vi "anglecalcs.vi"() -> ()   [LabVIEW 2015]
panel:
  out "thi6":dbl
  out "thi5":dbl
  out "thi4":dbl
  out "hyp2":dbl
  out "hyp1":dbl
  out "thi3":dbl
  out "thi2":dbl
  out "thi1":dbl
  out "h2":dbl
  out "h1":dbl
  out "x2":dbl
  out "x1":dbl
  in  "start":dbl[](array[numeric])
  in  "Finish":dbl[](array[numeric])
  in  "laser":dbl[](array[numeric])
  in  "laser height":dbl
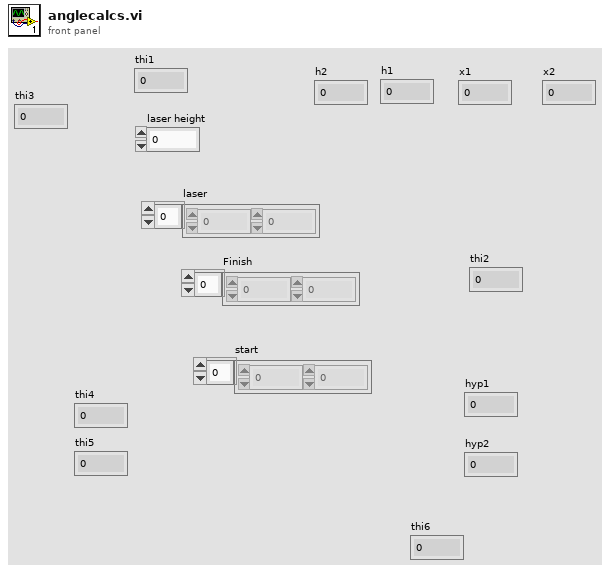
[diagram p1: front panel]
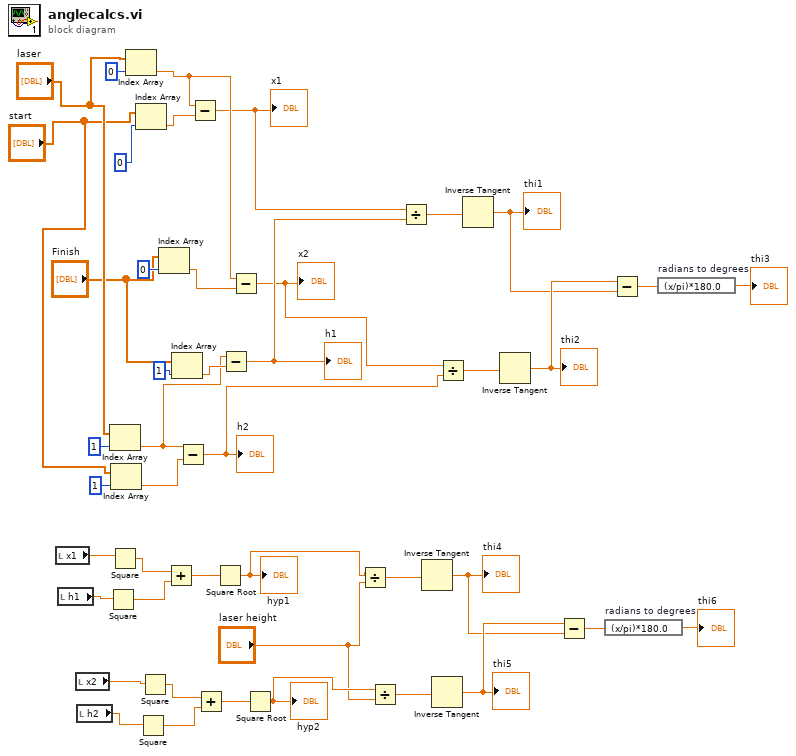
[diagram p0: block diagram]
diagram:
  n1 = local read "x1"() -> (w18:dbl)
  n2 = local read "h1"() -> (w19:dbl)
  n3 = local read "x2"() -> (w11:dbl)
  n4 = local read "h2"() -> (w10:dbl)
  n5 = Square(x=w19) -> (x^2=w16:dbl)
  n6 = Index Array(array="laser", index=1) -> (element=w30:dbl)
  n7 = Square(x=w18) -> (x^2=w17:dbl)
  n8 = Index Array(array="start", index=1) -> (element=w33:dbl)
  n9 = Index Array(array="laser", index=0) -> (element=w41:dbl)
  n10 = Index Array(array="start", index=0) -> (element=w40:dbl)
  n11 = Square(x=w10) -> (x^2=w13:dbl)
  n12 = Square(x=w11) -> (x^2=w14:dbl)
  n13 = Index Array(array="Finish", index=0) -> (element=w39:dbl)
  n14 = Add(x=w17, y=w16) -> (x+y=w15:dbl)
  n15 = Index Array(array="Finish", index=1) -> (element=w32:dbl)
  n16 = Subtract(x=w30, y=w33) -> (x-y=w24:dbl)
  "h2" <- w24
  n17 = Subtract(x=w41, y=w40) -> (x-y=w28:dbl)
  "x1" <- w28
  n18 = Add(x=w14, y=w13) -> (x+y=w12:dbl)
  n19 = Square Root(x=w15) -> (sqrt(x)=w8:dbl)
  "hyp1" <- w8
  n20 = Subtract(x=w30, y=w32) -> (x-y=w29:dbl)
  "h1" <- w29
  n21 = Subtract(x=w41, y=w39) -> (x-y=w25:dbl)
  "x2" <- w25
  n22 = Square Root(x=w12) -> (sqrt(x)=w6:dbl)
  "hyp2" <- w6
  n23 = Divide(x=w8, y="laser height") -> (x/y=w9:dbl)
  n24 = Divide(x=w6, y="laser height") -> (x/y=w7:dbl)
  n25 = Divide(x=w28, y=w29) -> (x/y=w27:dbl)
  n26 = Inverse Tangent(1:w9) -> (0:w1:dbl)
  "thi4" <- w1
  n27 = Inverse Tangent(1:w7) -> (0:w2:dbl)
  "thi5" <- w2
  n28 = Divide(x=w25, y=w24) -> (x/y=w26:dbl)
  n29 = Inverse Tangent(1:w27) -> (0:w22:dbl)
  "thi1" <- w22
  n30 = Inverse Tangent(1:w26) -> (0:w23:dbl)
  "thi2" <- w23
  n31 = Subtract(x=w2, y=w1) -> (x-y=w3:dbl)
  n32 = expression code="(x/pi)*180.0" "radians to degrees"(w3) -> (→"thi6":dbl)
  n33 = Subtract(x=w23, y=w22) -> (x-y=w20:dbl)
  n34 = expression code="(x/pi)*180.0" "radians to degrees"(w20) -> (→"thi3":dbl)
